vi "DAQ AO inventory (SubVI).vi"(7 "Use DAQ AO?":bool[](array[boolean]), 8 "error in (no error)":errorcluster, 9 "Address in":tag[](array[tag]), 10 "Max":dbl[](array[numeric]), 11 "Min":dbl[](array[numeric])) -> (0 "error out":errorcluster, 2 "Address out":refnum<k21>[](array[refnum]), 3 "DAQ names out":string[](array[string]))   [LabVIEW 2025, in "MyDaq.lvlib"]
uses:
  MyDaq.lvlib
  <vilib>/DAQmx/create/channels.llb/DAQmx Create Channel (AO-Voltage-Basic).vi
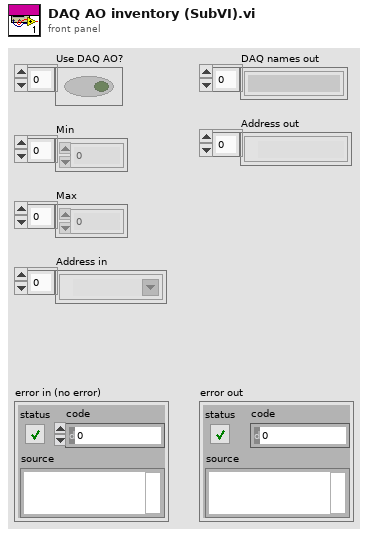
[diagram p1: front panel]
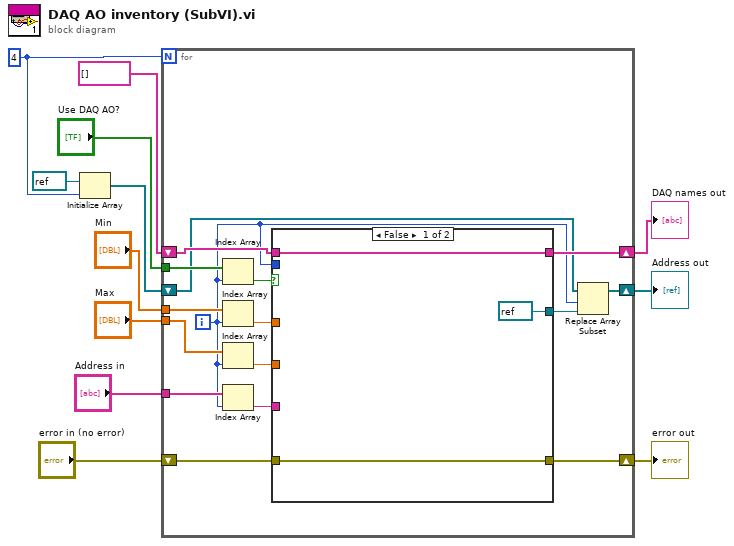
[diagram p0: block diagram]
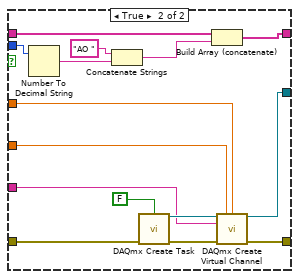
[diagram p2: hidden frame]
diagram:
  w3 = 4
  n1 = Initialize Array(refnum<k21> refnum ("task out"), w3) -> (w4:refnum<k21>[])
  n2 = for {
    N: w3 -> [_]
    tunnel: "Address in" -> [w18]
    tunnel: "Min" -> [w22]
    tunnel: "Max" -> [w20]
    shift-right: [w27] -> w5
    shift-left: "error in (no error)" -> [w28]
    tunnel: "Use DAQ AO?" -> [w24]
    shift-right: [w15] -> w7
    shift-left: w4 -> [w14]
    shift-right: [w26] -> w11
    shift-left: string[] [] ("DAQ names in") -> [w25]
    i -> [w13]
    n3 = Index Array(array=w24, index=w13) -> (element=w23:bool)
    n4 = Index Array(array=w22, index=w13) -> (element=w21:dbl)
    n5 = Index Array(array=w20, index=w13) -> (element=w19:dbl)
    n6 = Index Array(array=w18, index=w13) -> (element=w17:tag)
    n7 = case shown="False" w23 {
      tunnel: w17 -> [_ w43]
      tunnel: [refnum<k21> refnum ("task out") w42] -> w16
      tunnel: w21 -> [_ w41]
      tunnel: w19 -> [_ w40]
      tunnel: w28 -> [w31 w39]
      tunnel: [w31 w38] -> w27
      tunnel: [w29 w36] -> w26
      tunnel: w25 -> [w29 w37]
      tunnel: w13 -> [_ w33]
      frame False {
      }
      frame True {
        n8 = Number To Decimal String(number=w33) -> (decimal integer string=w32:string)  [unwired: 1 in]
        n9 = Concatenate Strings("AO " ("string"), w32) -> (w35:string)
        n10 = call <vilib>:"DAQmx Create Task.vi"("auto cleanup"=FALSE, "error in"=w39) -> ("task out"=w45:refnum<k21>, "error out"=w44:errorcluster)  [unwired: 12 in]
        n11 = Build Array (concatenate)(w37, w35) -> (w36:string[])
        n12 = call-poly <vilib>:"DAQmx Create Virtual Channel.vi"("task in"=w45, "maximum value"=w40, "minimum value"=w41, "physical channels"=w43, "error in"=w44) -> ("task out"=w42:refnum<k21>, "error out"=w38:errorcluster)  [unwired: 9 in]
      }
    }
    n13 = Replace Array Subset(array=w14, new element=w16, index=w13) -> (w15:refnum<k21>[])
  }
  "DAQ names out" <- w11
  "Address out" <- w7
  "error out" <- w5
